vi "OPC Test.vi"() -> ()   [LabVIEW 2015]
uses:
  Library/Shot data.ctl
panel:
  out "Shot data":T1
  out "Data Ready":bool
  in  "Data URL 2":string="opc:\\cyberlogic.opcserverDA\\UB.DataReady"
  out "timed out":bool
  out "quality":u64 format="%b"
  out "status":u32
  out "string":string
  out "data 5":u16[](array[numeric])
  out "data 4":string
  out "data 3":bool
  out "data 2":i16
  out "data":sgl
  in  "Type":T2(ring)=enum."INT ARRAY"
  out "Variant":variant
  in  "Data URL":string="opc:\\cyberlogic.opcserverDA\\UB.MagHistString"
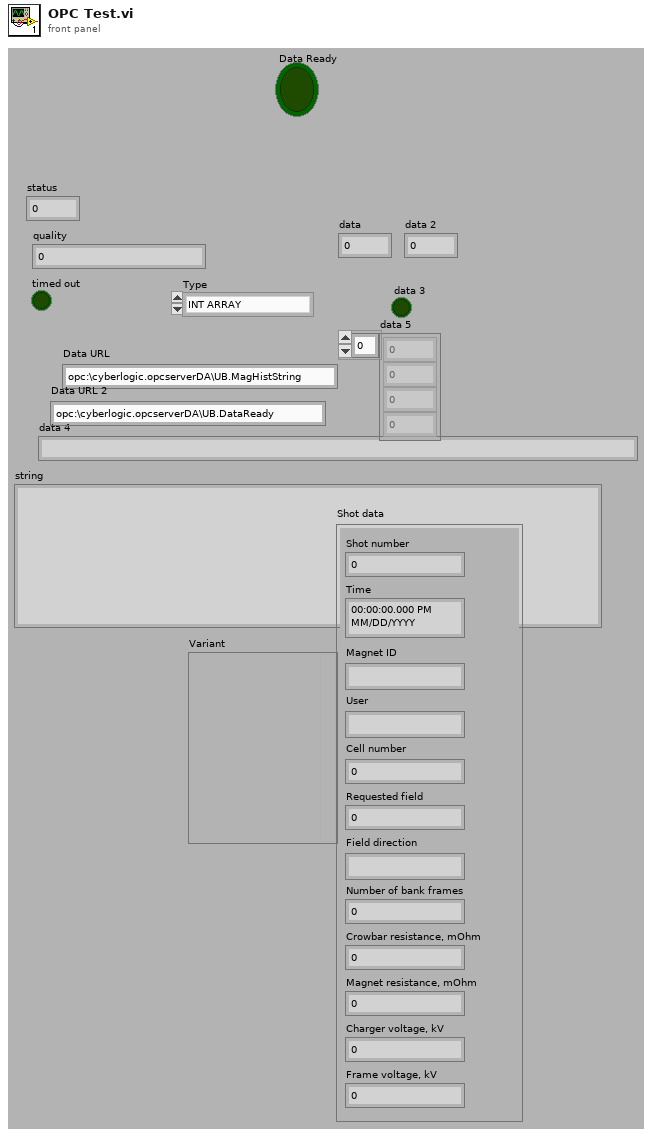
[diagram p1: front panel]
types:
  T1 = typedef "Shot data.ctl" = cluster{"Shot number":i32, "Time":timestamp, "Magnet ID":string, "User":string, "Cell number":i32, "Requested field":dbl, "Field direction":string, "Number of bank frames":i32, "Crowbar resistance, mOhm":dbl, "Magnet resistance, mOhm":dbl, "Charger voltage, kV":dbl, "Frame voltage, kV":dbl}
  T2 = enum16{"FLOAT", "ASCII", "INT", "INT ARRAY", "BOOL"}
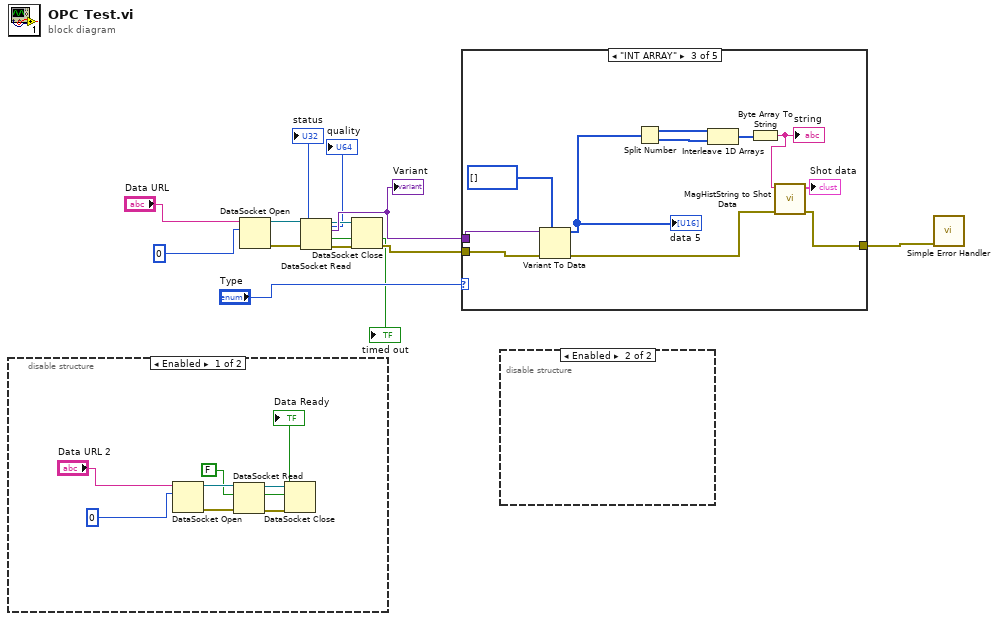
[diagram p0: block diagram]
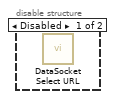
[diagram p2: hidden frame]
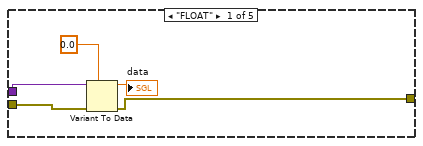
[diagram p4: hidden frame]
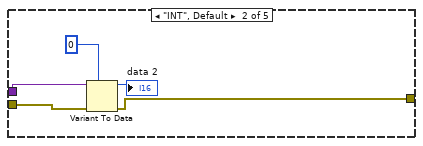
[diagram p5: hidden frame]
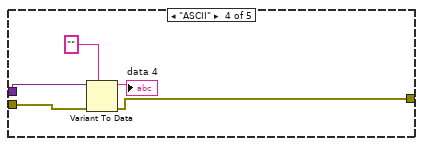
[diagram p6: hidden frame]
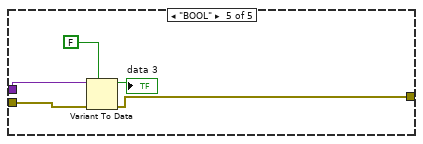
[diagram p7: hidden frame]
diagram:
  n1 = disable-structure shown="Enabled" {
    frame Enabled {
      n2 = DataSocket Open(10:0, 11:"Data URL 2") -> (0:w18:errorcluster, 3:w20:refnum<k13>)  [unwired: 2 in]
      n3 = DataSocket Read(8:w18, 10:FALSE, 11:w20) -> (0:w17:errorcluster, 2:→"Data Ready":bool, 3:w16:refnum<k13>)  [unwired: 2 in, 4 out]
      n4 = DataSocket Close(8:w17, 11:w16) -> ()  [unwired: 1 in, 2 out]
    }
    frame Disabled {
    }
  }
  n5 = DataSocket Open(10:0, 11:"Data URL") -> (0:w10:errorcluster, 3:w12:refnum<k13>)  [unwired: 2 in]
  n6 = DataSocket Read(8:w10, 11:w12) -> (0:w6:errorcluster, 1:→"timed out":bool, 2:w8:variant, 3:w5:refnum<k13>, 5:→"quality":u64, 7:→"status":u32)  [unwired: 3 in, 1 out]
  "Variant" <- w8
  n7 = DataSocket Close(8:w6, 11:w5) -> (0:w4:errorcluster)  [unwired: 1 in, 1 out]
  n8 = case shown="\"INT ARRAY\"" "Type" {
    tunnel: w8 -> [w26 w31 w42 w47 w52]
    tunnel: w4 -> [w25 w30 w41 w46 w51]
    tunnel: [w24 w29 w32 w45 w50] -> w7
    frame "FLOAT" {
      n9 = Variant To Data(error in=w25, type=sgl 0.0, Variant=w26) -> (data=→"data":sgl, error out=w24:errorcluster)
    }
    frame "INT", Default {
      n10 = Variant To Data(error in=w30, type=i16 0, Variant=w31) -> (data=→"data 2":i16, error out=w29:errorcluster)
    }
    frame "INT ARRAY" {
      n11 = Variant To Data(error in=w41, type=u16[] [], Variant=w42) -> (data=w39:u16[], error out=w33:errorcluster)
      "data 5" <- w39
      n12 = Split Number(x=w39) -> (hi(x)=w38:u8[], lo(x)=w37:u8[])
      n13 = Interleave 1D Arrays(w38, w37) -> (w36:u8[])
      n14 = Byte Array To String(unsigned byte array=w36) -> (string=w35:string)
      "string" <- w35
      n15 = call "MagHistString to Shot Data.vi"("error in (no error)"=w33, "String"=w35) -> ("error out"=w32:errorcluster, "Shot data"=→"Shot data":T1)  [unwired: 8 in]
    }
    frame "ASCII" {
      n16 = Variant To Data(error in=w46, type="", Variant=w47) -> (data=→"data 4":string, error out=w45:errorcluster)
    }
    frame "BOOL" {
      n17 = Variant To Data(error in=w51, type=FALSE, Variant=w52) -> (data=→"data 3":bool, error out=w50:errorcluster)
    }
  }
  n18 = disable-structure shown="Enabled" {
    frame Disabled {
      n19 = call <vilib>:"DataSocket Select URL.vi"() -> ()  [unwired: 9 in, 3 out]
    }
    frame Enabled {
    }
  }
  n20 = call <vilib>:"Simple Error Handler.vi"("error in (no error)"=w7) -> ()  [unwired: 4 in, 5 out]
